vi "High Precision AT Data.vi"(11 "Cluster":T1) -> (3 "String":string)   [LabVIEW 2019, in "Acquisition.lvlib"]
uses:
  Acquisition/Acquisition.lvlib
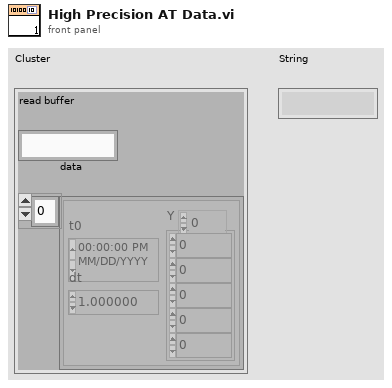
[diagram p1: front panel]
types:
  T1 = cluster{"read buffer":string, "data":waveform(dbl)[]}
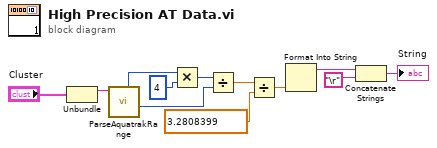
[diagram p0: block diagram]
diagram:
  n1 = Unbundle("Cluster") -> ("read buffer"=w2:string)  [unwired: 1 out]
  n2 = call "ParseAquatrakRange.vi"("Incoming String"=w2) -> ("Cal Counts"=w3:i32, "Range Counts"=w4:i32)  [unwired: 6 in, 3 out]
  n3 = Multiply(x=w4, y=4) -> (x*y=w6:i32)
  n4 = Divide(x=w6, y=w3) -> (x/y=w10:dbl)
  n5 = Divide(x=w10, y=3.2808399) -> (x/y=w11:dbl)
  n6 = Format Into String(w11) -> (resulting string=w9:string)  [unwired: 3 in, 1 out]
  n7 = Concatenate Strings(w9, "\r") -> (→"String":string)
